vi "ParseNumber.vi"(8 "error in (no error)":errorcluster, 10 "Index In":i32, 11 "JSON String":string) -> (0 "error out":errorcluster, 2 "Index Out":i32, 3 "JSON Tree":variant)   [LabVIEW 2013, in "i3-json.lvlib"]
doc: "Use this template to build a VI to use as a subVI."
uses:
  i3-json.lvlib
  JSON Types/JSON Type.ctl
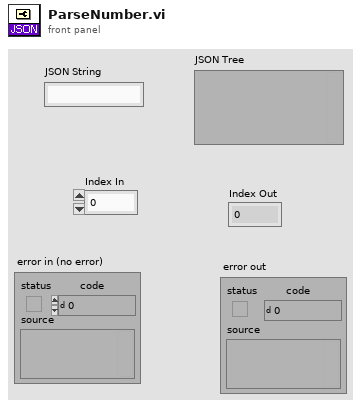
[diagram p1: front panel]
types:
  T1 = typedef "i3-json.lvlib/JSON Type.ctl" = enum8{"JSON Compatible", "JSON Array", "JSON Object", "JSON Null", "Double", "String", "Boolean", "Unknown", "Data JSON string"}
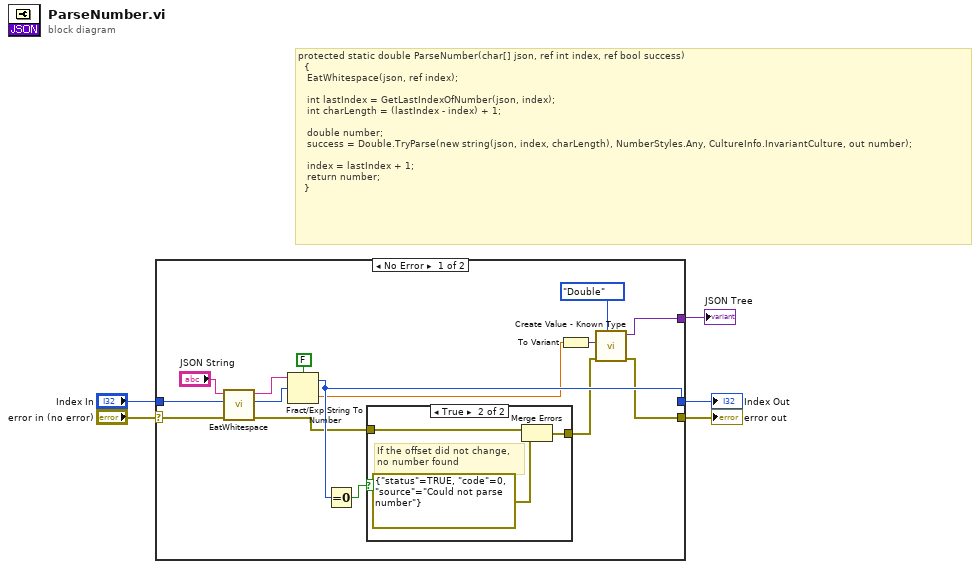
[diagram p0: block diagram]
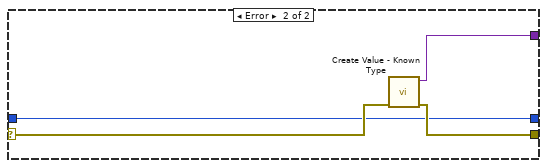
[diagram p3: hidden frame]
diagram:
  # "protected static double ParseNumber(char[] json, ref int index, ref bool success)\n\t\t{\n\t\t\tEatWhitespace(json, ref index);\n\n\t\t\tint lastIndex = GetLastIndexOfNumber(json, index);\n\t\t\tint charLength = (lastIndex - index) + 1;\n\n\t\t\tdouble number;\n\t\t\tsuccess = Double.TryParse(new string(json, index, charLength), NumberStyles.Any, CultureInfo.InvariantCulture, out number);\n\n\t\t\tindex = lastIndex + 1;\n\t\t\treturn number;\n\t\t}"
  n1 = case shown="No Error" "error in (no error)" {
    selector: "error in (no error)" -> [w18 w27]
    tunnel: [w14 w28] -> w4
    tunnel: [w13 w26] -> w3
    tunnel: "Index In" -> [w19 w25]
    tunnel: [w15 w25] -> w1
    frame No Error {
      n2 = call "EatWhitespace.vi"("error in (no error)"=w18, "Index In"=w19, "JSON String"="JSON String") -> ("error out"=w8:errorcluster, "Index Out"=w16:i32, "JSON String Passthrough"=w17:string)  [unwired: 6 in]
      n3 = Fract/Exp String To Number(use system decimal point (T)=FALSE, string=w17, offset=w16) -> (offset past number=w15:i32, number=w10:dbl)  [unwired: 1 in]
      n4 = Equal To 0?(x=w15) -> (x = 0?=w9:bool)
      n5 = case shown="True" w9 {
        tunnel: w8 -> [w21 w24]
        tunnel: [w21 w22] -> w7
        frame False {
        }
        frame True {
          # "If the offset did not change,\nno number found"
          n6 = Merge Errors(w24, errorcluster {"status"=TRUE, "code"=0, "source"="Could not parse number"} ("t")) -> (w22:errorcluster)
        }
      }
      n7 = To Variant(anything=w10) -> (Variant=w11:variant)
      n8 = call "Create Value - Known Type.vi"("JSON Type"=JSON_Type."Double", "error in (no error)"=w7, "Value"=w11) -> ("error out"=w14:errorcluster, "JSON Tree"=w13:variant)  [unwired: 7 in]
    }
    frame Error {
      n9 = call "Create Value - Known Type.vi"("error in (no error)"=w27) -> ("error out"=w28:errorcluster, "JSON Tree"=w26:variant)  [unwired: 9 in]
    }
  }
  "error out" <- w4
  "Index Out" <- w1
  "JSON Tree" <- w3
